vi "Analog Input DAQ Engine.vi"(8 "error in":errorcluster, 10 "DAQ Engine":refnum<notifier>, 11 "Sequence Context In":refnum<k7>) -> (0 "error out":errorcluster)   [LabVIEW 2023, in "LTT_TeststandSteptypes.lvlib"]
uses:
  LTT_TeststandSteptypes.lvlib
  HardwareAbstractionLayer_LVOOP/Analog Input/NI Analog Input/NI Analog Input.lvclass
  D:/eDCU LTT/VT LTT Project/Source Code/HardwareAbstractionLayer_LVOOP/Analog Input/AI/AI.lvclass
  HardwareAbstractionLayer_LVOOP/Main/Class Ref.ctl
  HardwareAbstractionLayer_LVOOP/DMM/DMM.lvclass
  HardwareAbstractionLayer_LVOOP/Function Generator/Function Generator.lvclass
  HardwareAbstractionLayer_LVOOP/Oscilloscope/Oscilloscope.lvclass
  HardwareAbstractionLayer_LVOOP/PowerSupply/PowerSupply.lvclass
  HardwareAbstractionLayer_LVOOP/Teststand/Teststand.lvclass
  HardwareAbstractionLayer_LVOOP/Analog Output/AO/AO.lvclass
  HardwareAbstractionLayer_LVOOP/Analog Input/AI/AI.lvclass
  HardwareAbstractionLayer_LVOOP/Database/Database.lvclass
  HardwareAbstractionLayer_LVOOP/Digital Output/DO_class/DO.lvclass
  HardwareAbstractionLayer_LVOOP/Digital Input/DI_class/DI.lvclass
  HardwareAbstractionLayer_LVOOP/PWM Output/PWM Output_class/PWM Output.lvclass
  HardwareAbstractionLayer_LVOOP/PWM Input/PWM Input_class/PWM Input.lvclass
  HardwareAbstractionLayer_LVOOP/NI Switch/NISwitch_class/NISwitch.lvclass
  HardwareAbstractionLayer_LVOOP/Modbus/Modbus_class/Modbus.lvclass
  HardwareAbstractionLayer_LVOOP/CAN/CAN Lib/CAN_class/CAN.lvclass
  HardwareAbstractionLayer_LVOOP/Main/Class Options.ctl
  <vilib>/Utility/error.llb/DialogType.ctl
  HardwareAbstractionLayer_LVOOP/Main/Main.lvclass
panel:
  in  "stop":bool
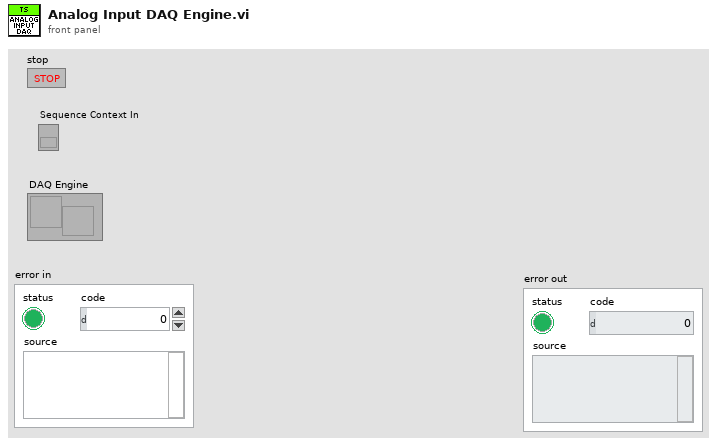
[diagram p1: front panel]
types:
  T1 = typedef "HardwareAbstractionLayer_LVOOP.lvlib/Main.lvclass/Class Ref.ctl" = cluster{"DMM":refnum<class "DMM.lvclass">, "Function Generator":refnum<class "Function Generator.lvclass">, "Oscilloscope":refnum<class "Oscilloscope.lvclass">, "PowerSupply":refnum<class "PowerSupply.lvclass">, "Teststand":refnum<class "Teststand.lvclass">, "AO":refnum<class "AO.lvclass">, "AI":refnum<class "AI.lvclass">, "Database":refnum<class "Database.lvclass">, "AO Waveform Generation":refnum<class "AO.lvclass">, "DO":refnum<class "DO.lvclass">, "DI":refnum<class "DI.lvclass">, "PWM Output":refnum<class "PWM Output.lvclass">, "PWM Input":refnum<class "PWM Input.lvclass">, "RelayOutput":refnum<class "NISwitch.lvclass">, "Modbus":refnum<class "Modbus.lvclass">, "CAN":refnum<class "CAN.lvclass">}
  T2 = typedef "HardwareAbstractionLayer_LVOOP.lvlib/Main.lvclass/Class Options.ctl" = enum16{"Init All Class", "Read All Class", "Write AI Class", "Write AO Class", "Write AO Waveform Generation", "Write DI Class", "Write DO Class", "Write PWM Input Class", "Write PWM Output Class", "Exit"}
  T3 = typedef "DialogType.ctl" = u16
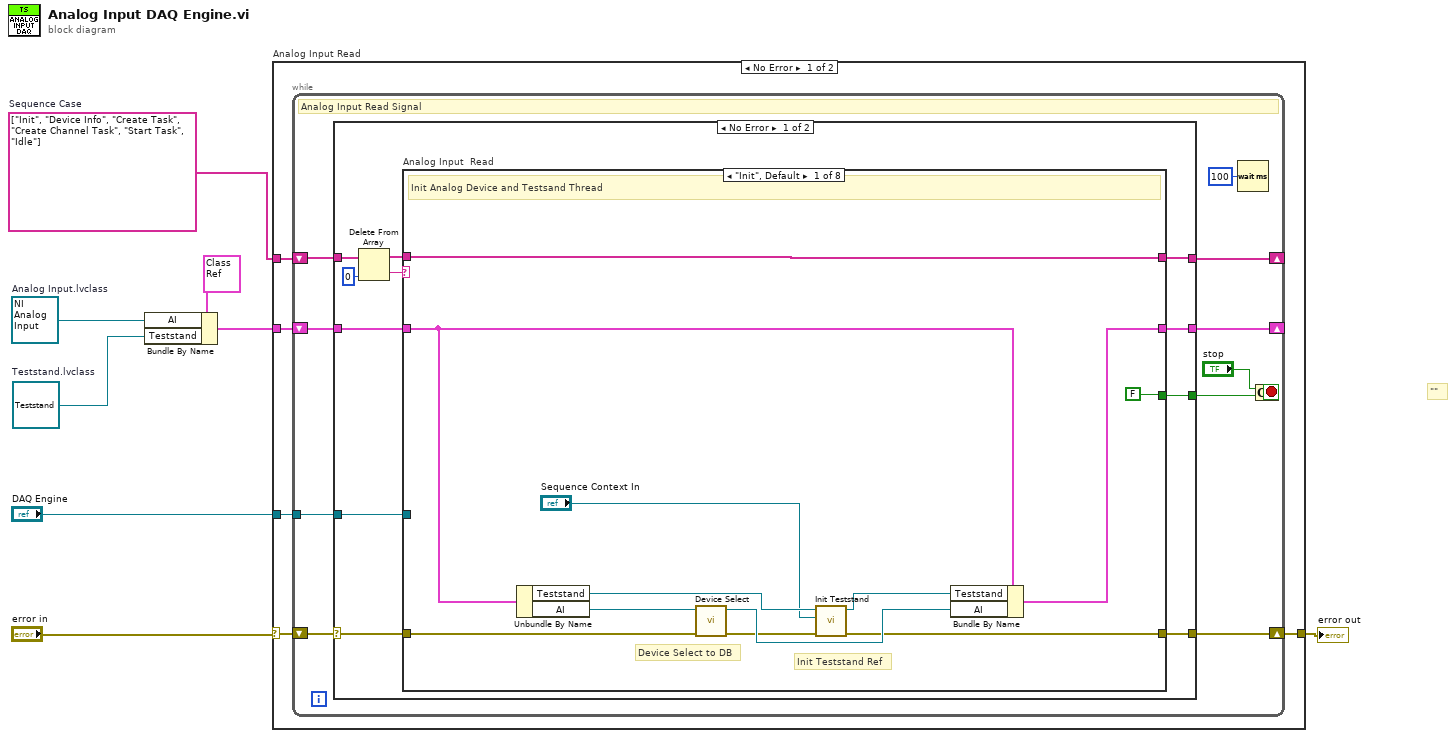
[diagram p0: block diagram]
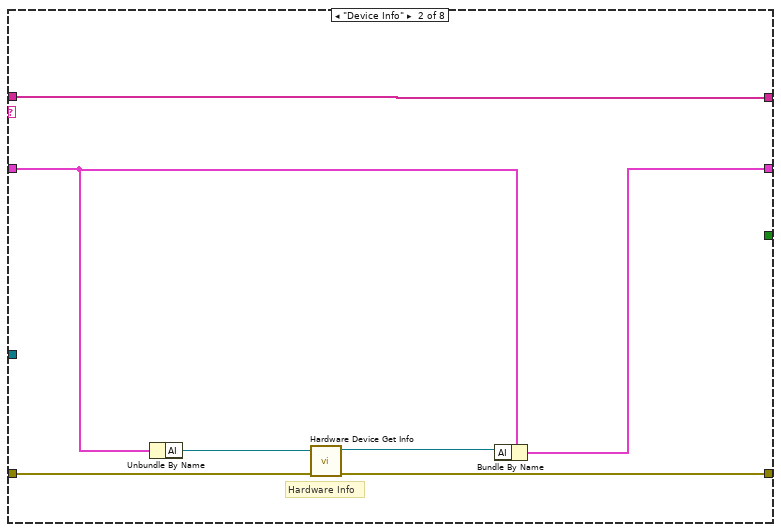
[diagram p2: hidden frame]
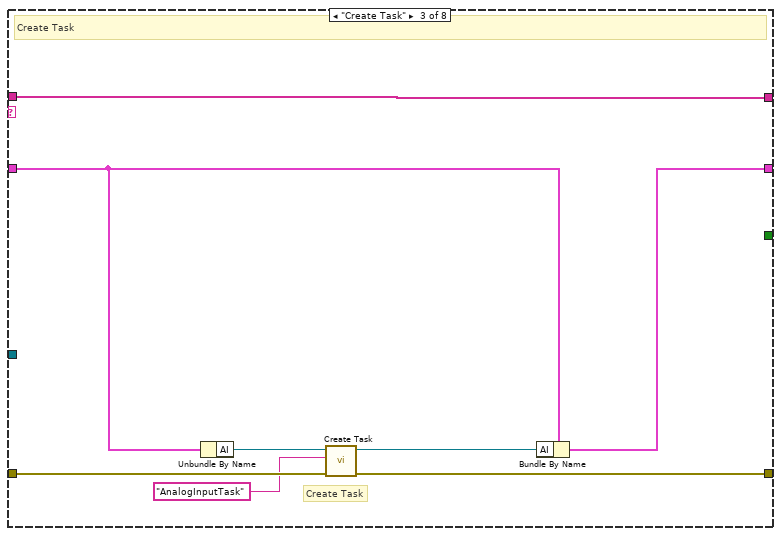
[diagram p3: hidden frame]
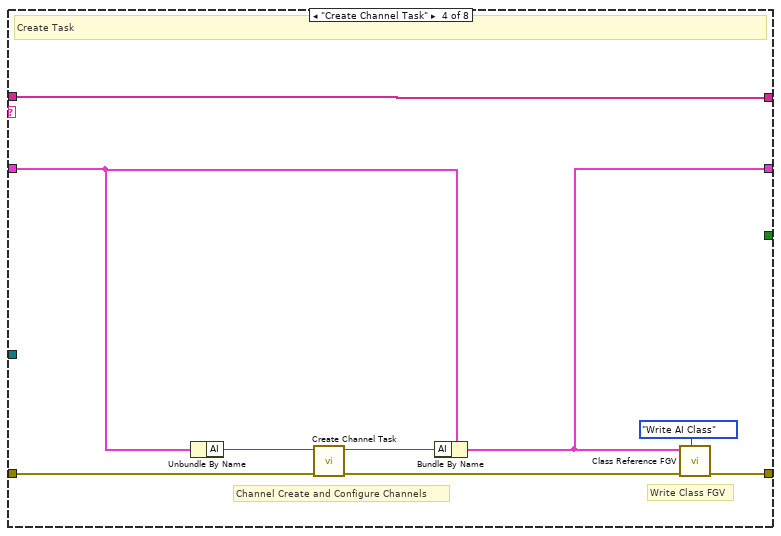
[diagram p4: hidden frame]
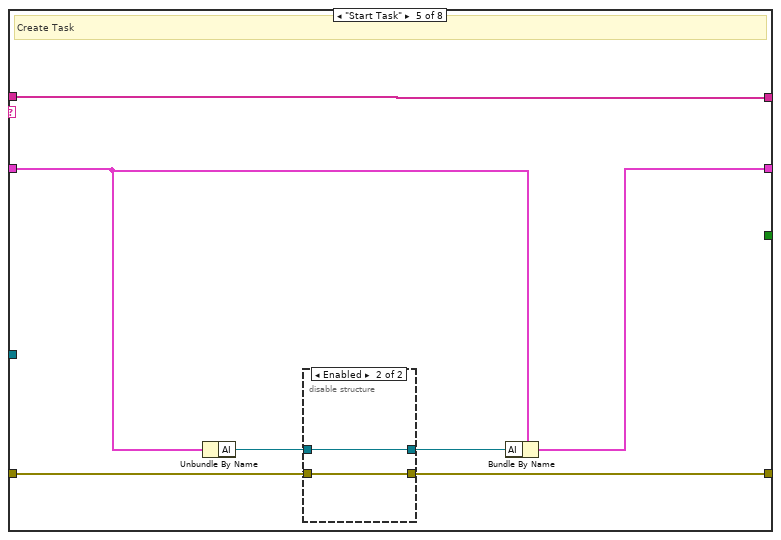
[diagram p5: hidden frame]
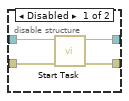
[diagram p6: hidden frame]
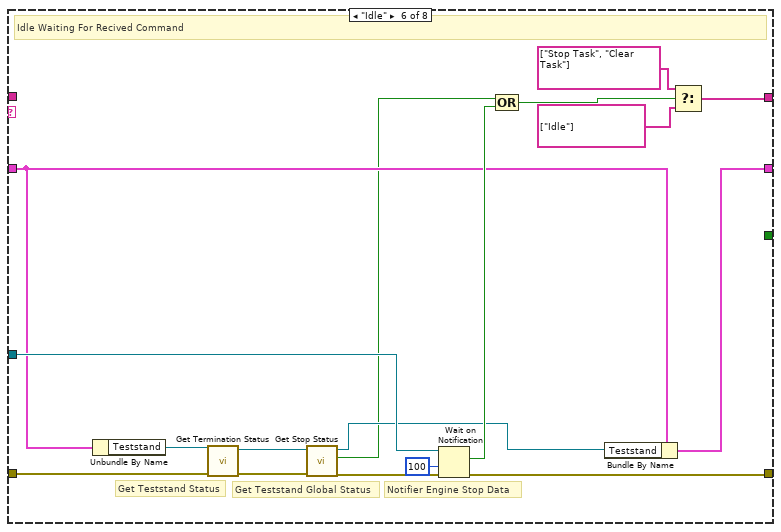
[diagram p7: hidden frame]
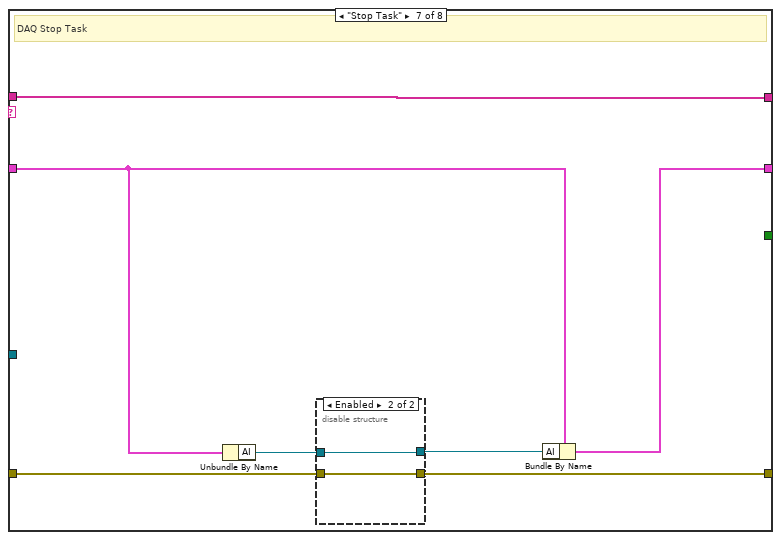
[diagram p8: hidden frame]
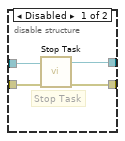
[diagram p9: hidden frame]
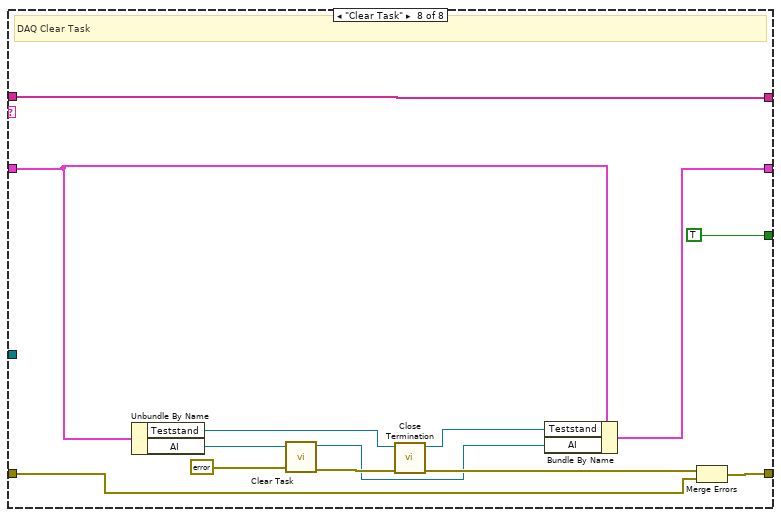
[diagram p10: hidden frame]
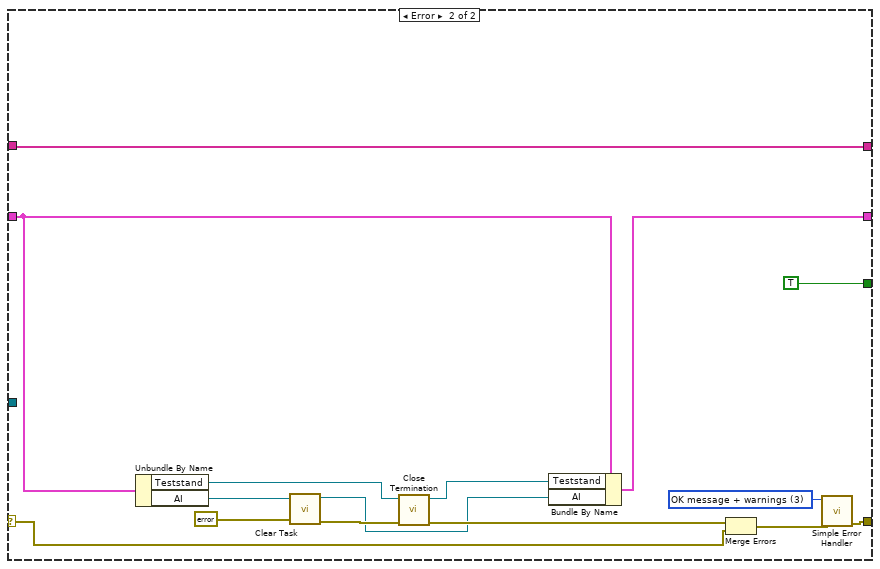
[diagram p11: hidden frame]
diagram:
  w1 = refnum<class "Teststand.lvclass"> refnum  # Teststand.lvclass
  w3 = string[] ["Init", "Device Info", "Create Task", "Create Channel Task", "Start Task", "Idle"]  # Sequence Case
  w5 = refnum<class "NI Analog Input.lvclass"> refnum  # Analog Input.lvclass
  # "\"\""
  n1 = Bundle By Name(cluster=T1 {"DMM"=refnum, "Function Generator"=refnum, "Oscilloscope"=refnum, "PowerSupply"=refnum, "Teststand"=refnum, "AO"=refnum, "AI"=refnum, "Database"=refnum, "AO Waveform Generation"=refnum, "DO"=refnum, "DI"=refnum, "PWM Output"=refnum, "PWM Input"=refnum, "RelayOutput"=refnum, "Modbus"=refnum, "CAN"=refnum} ("Class Cluster"), "AI"=w5, "Teststand"=w1) -> (w4:T1)
  n2 = case "Analog Input Read" shown="No Error" "error in" {
    selector: "error in" -> [w13 w143]
    tunnel: [w12 w143] -> w7
    tunnel: w4 -> [w11 _]
    tunnel: w3 -> [w10 _]
    tunnel: "DAQ Engine" -> [w9 _]
    frame No Error {
      n3 = while {
        shift-right: [w23] -> w12
        shift-left: w13 -> [w24]
        shift-right: [w21] -> _
        shift-left: w11 -> [w22]
        shift-right: [w19] -> _
        shift-left: w10 -> [w20]
        tunnel: w9 -> [w14]
        stop <- w16 stop-if-true
        # "Analog Input Read Signal"
        n4 = case shown="No Error" w24 {
          selector: w24 -> [w35 w132]
          tunnel: [w34 w129] -> w23
          tunnel: w22 -> [w30 w134]
          tunnel: [w29 w133] -> w21
          tunnel: w20 -> [w33 w131]
          tunnel: [w27 w131] -> w19
          tunnel: [w26 TRUE] -> w15
          tunnel: w14 -> [w25 _]
          frame No Error {
            n5 = Delete From Array(array=w33, index=0) -> (deleted portion=w32:string, array with subset deleted=w28:string[])  [unwired: 1 in]
            n6 = case "Analog Input  Read" shown="\"Init\", Default" w32 {
              tunnel: w35 -> [w44 w52 w57 w69 w75 w90 w105 w116]
              tunnel: [w38 w51 w56 w65 w74 w96 w104 w117] -> w34
              tunnel: w30 -> [w46 w50 w61 w70 w77 w93 w107 w126]
              tunnel: [w45 w49 w60 w64 w76 w92 w106 w125] -> w29
              tunnel: w28 -> [w47 w54 w62 w71 w78 _ w108 w127]
              tunnel: [w47 w54 w62 w71 w78 w99 w108 w127] -> w27
              tunnel: [FALSE _ _ _ _ _ _ TRUE] -> w26
              tunnel: w25 -> [_ _ _ _ _ w97 _ _]
              frame "Init", Default {
                # "Init Teststand Ref"
                # "Device Select to DB"
                # "Init Analog Device and Testsand Thread"
                n7 = Unbundle By Name(w46) -> ("Teststand"=w40:refnum<class "Teststand.lvclass">, "AI"=w41:refnum<class "AI.lvclass">)
                n8 = call-dynamic "Device Select.vi"("error in (no error)"=w44, "AI in"=w41) -> ("error out"=w39:errorcluster, "AI out"=w43:refnum<class "AI.lvclass">)  [unwired: 8 in]
                n9 = call-dynamic "Init Teststand.vi"("error in (no error)"=w39, "Sequence Context In"="Sequence Context In", "Teststand in"=w40) -> ("error out"=w38:errorcluster, "Teststand out"=w37:refnum<class "Teststand.lvclass">)  [unwired: 7 in]
                n10 = Bundle By Name(cluster=w46, "Teststand"=w37, "AI"=w43) -> (w45:T1)
              }
              frame "Device Info" {
                # "Hardware Info"
                n11 = Unbundle By Name(w50) -> ("AI"=w53:refnum<class "AI.lvclass">)
                n12 = call-dynamic "Hardware Device Get Info.vi"("error in (no error)"=w52, "AI in"=w53) -> ("error out"=w51:errorcluster, "AI out"=w48:refnum<class "AI.lvclass">)  [unwired: 8 in]
                n13 = Bundle By Name(cluster=w50, "AI"=w48) -> (w49:T1)
              }
              frame "Create Task" {
                # "Create Task"
                # "Create Task"
                n14 = Unbundle By Name(w61) -> ("AI"=w59:refnum<class "AI.lvclass">)
                n15 = call-dynamic "Create Task.vi"("error in (no error)"=w57, "Task name"="AnalogInputTask", "AI in"=w59) -> ("error out"=w56:errorcluster, "AI out"=w58:refnum<class "AI.lvclass">)  [unwired: 7 in]
                n16 = Bundle By Name(cluster=w61, "AI"=w58) -> (w60:T1)
              }
              frame "Create Channel Task" {
                # "Write Class FGV"
                # "Channel Create and Configure Channels"
                # "Create Task"
                n17 = Unbundle By Name(w70) -> ("AI"=w68:refnum<class "AI.lvclass">)
                n18 = call-dynamic "Create Channel Task.vi"("error in (no error)"=w69, "AI in"=w68) -> ("error out"=w66:errorcluster, "AI out"=w67:refnum<class "AI.lvclass">)  [unwired: 8 in]
                n19 = Bundle By Name(cluster=w70, "AI"=w67) -> (w64:T1)
                n20 = call "Class Reference FGV.vi"("Options"=Class_Options."Write AI Class", "error in"=w66, "Class Cluster In"=w64) -> ("error out"=w65:errorcluster)  [unwired: 7 in, 1 out]
              }
              frame "Start Task" {
                # "Create Task"
                n21 = Unbundle By Name(w77) -> ("AI"=w73:refnum<class "AI.lvclass">)
                n22 = disable-structure shown="Enabled" {
                  disable-tunnel: w75 -> [w82 w84]
                  disable-tunnel: [w81 w84] -> w74
                  disable-tunnel: w73 -> [w80 w83]
                  disable-tunnel: [w79 w83] -> w72
                  frame Disabled {
                    n23 = call-dynamic "Start Task.vi"("error in (no error)"=w82, "AI in"=w80) -> ("error out"=w81:errorcluster, "AI out"=w79:refnum<class "AI.lvclass">)  [unwired: 8 in]
                  }
                  frame Enabled {
                  }
                }
                n24 = Bundle By Name(cluster=w77, "AI"=w72) -> (w76:T1)
              }
              frame "Idle" {
                # "Notifier Engine Stop Data"
                # "Get Teststand Global Status"
                # "Get Teststand Status"
                # "Idle Waiting For Recived Command"
                n25 = Unbundle By Name(w93) -> ("Teststand"=w91:refnum<class "Teststand.lvclass">)
                n26 = call-dynamic "Get Termination Status.vi"("error in (no error)"=w90, "Teststand in"=w91) -> ("error out"=w89:errorcluster, "Teststand out"=w88:refnum<class "Teststand.lvclass">)  [unwired: 7 in, 1 out]
                n27 = call-dynamic "Get Stop Status.vi"("error in (no error)"=w89, "Teststand in"=w88) -> ("error out"=w87:errorcluster, "Value"=w85:bool, "Teststand out"=w86:refnum<class "Teststand.lvclass">)  [unwired: 7 in]
                n28 = Wait on Notification(notifier=w97, timeout in ms (-1)=100, error in (no error)=w87) -> (notification=w94:bool, error out=w96:errorcluster)  [unwired: 1 in, 2 out]
                n29 = Compound Arithmetic op=OR(w85, w94) -> (w98:bool)
                n30 = Bundle By Name(cluster=w93, "Teststand"=w86) -> (w92:T1)
                n31 = Select(t=string[] ["Stop Task", "Clear Task"], s=w98, f=string[] ["Idle"]) -> (s? t:f=w99:string[])
              }
              frame "Stop Task" {
                # "DAQ Stop Task"
                n32 = Unbundle By Name(w107) -> ("AI"=w103:refnum<class "AI.lvclass">)
                n33 = disable-structure shown="Enabled" {
                  disable-tunnel: w105 -> [w112 w114]
                  disable-tunnel: [w111 w114] -> w104
                  disable-tunnel: w103 -> [w110 w113]
                  disable-tunnel: [w109 w113] -> w102
                  frame Disabled {
                    # "Stop Task"
                    n34 = call-dynamic "Stop Task.vi"("error in (no error)"=w112, "AI in"=w110) -> ("error out"=w111:errorcluster, "AI out"=w109:refnum<class "AI.lvclass">)  [unwired: 8 in]
                  }
                  frame Enabled {
                  }
                }
                n35 = Bundle By Name(cluster=w107, "AI"=w102) -> (w106:T1)
              }
              frame "Clear Task" {
                # "DAQ Clear Task"
                n36 = Unbundle By Name(w126) -> ("Teststand"=w122:refnum<class "Teststand.lvclass">, "AI"=w124:refnum<class "AI.lvclass">)
                n37 = call-dynamic "Clear Task.vi"("error in (no error)"=errorcluster {"status"=FALSE, "code"=0, "source"=""}, "AI in"=w124) -> ("error out"=w121:errorcluster, "AI out"=w118:refnum<class "AI.lvclass">)  [unwired: 8 in]
                n38 = call-dynamic "Close Termination.vi"("error in (no error)"=w121, "Teststand in"=w122) -> ("error out"=w120:errorcluster, "Teststand out"=w119:refnum<class "Teststand.lvclass">)  [unwired: 8 in]
                n39 = Bundle By Name(cluster=w126, "Teststand"=w119, "AI"=w118) -> (w125:T1)
                n40 = Merge Errors(w120, w116) -> (w117:errorcluster)
              }
            }
          }
          frame Error {
            w128 = T3 3 items=["no dialog", "OK message", "continue or stop message", "OK message + warnings", "continue/stop + warnings"] ("type of dialog (OK msg:1)")
            n41 = Unbundle By Name(w134) -> ("Teststand"=w140:refnum<class "Teststand.lvclass">, "AI"=w141:refnum<class "AI.lvclass">)
            n42 = call-dynamic "Clear Task.vi"("error in (no error)"=errorcluster {"status"=FALSE, "code"=0, "source"=""}, "AI in"=w141) -> ("error out"=w139:errorcluster, "AI out"=w136:refnum<class "AI.lvclass">)  [unwired: 8 in]
            n43 = call-dynamic "Close Termination.vi"("error in (no error)"=w139, "Teststand in"=w140) -> ("error out"=w138:errorcluster, "Teststand out"=w137:refnum<class "Teststand.lvclass">)  [unwired: 8 in]
            n44 = Bundle By Name(cluster=w134, "Teststand"=w137, "AI"=w136) -> (w133:T1)
            n45 = Merge Errors(w138, w132) -> (w130:errorcluster)
            n46 = call <vilib>:"Simple Error Handler.vi"("type of dialog (OK msg:1)"=w128, "error in (no error)"=w130) -> ("error out"=w129:errorcluster)  [unwired: 3 in, 4 out]
          }
        }
        n47 = Wait (ms)(milliseconds to wait=u32 100) -> ()  [unwired: 1 out]
        n48 = Compound Arithmetic op=OR("stop", w15) -> (w16:bool)
      }
    }
    frame Error {
      # "Error"
    }
  }
  "error out" <- w7
